vi "list energy peak.vi"() -> (1 "Energies Ordered":dbl[](array[numeric]), 2 "List Ordered":string[][](array[string]), 3 "List":string[][](array[string]))   [LabVIEW 2020]
uses:
  4b7d1e91-fce0-d643-892a-bcd5e833a70f.vi
  <vilib>/Utility/file.llb/Read Delimited Spreadsheet (string).vi
  <vilib>/Utility/Data Type/Get Array Information.vi
  <vilib>/Utility/Data Type/Get Type Information.vi
panel:
  out "appended array":string[][](array[string])
  out "list_peak_energies":string[][](array[string])
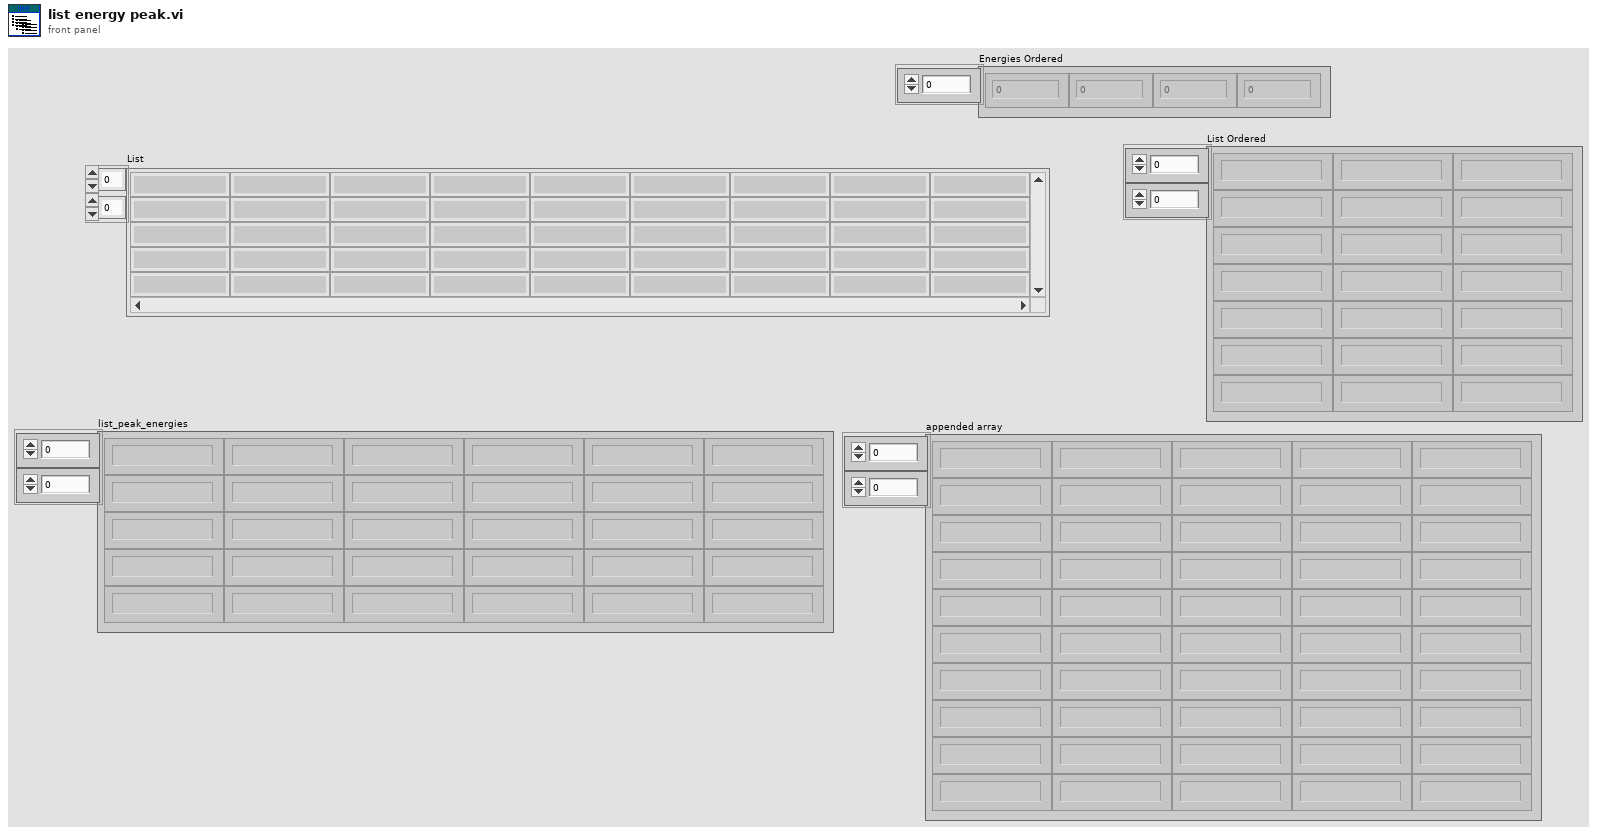
[diagram p1: front panel]
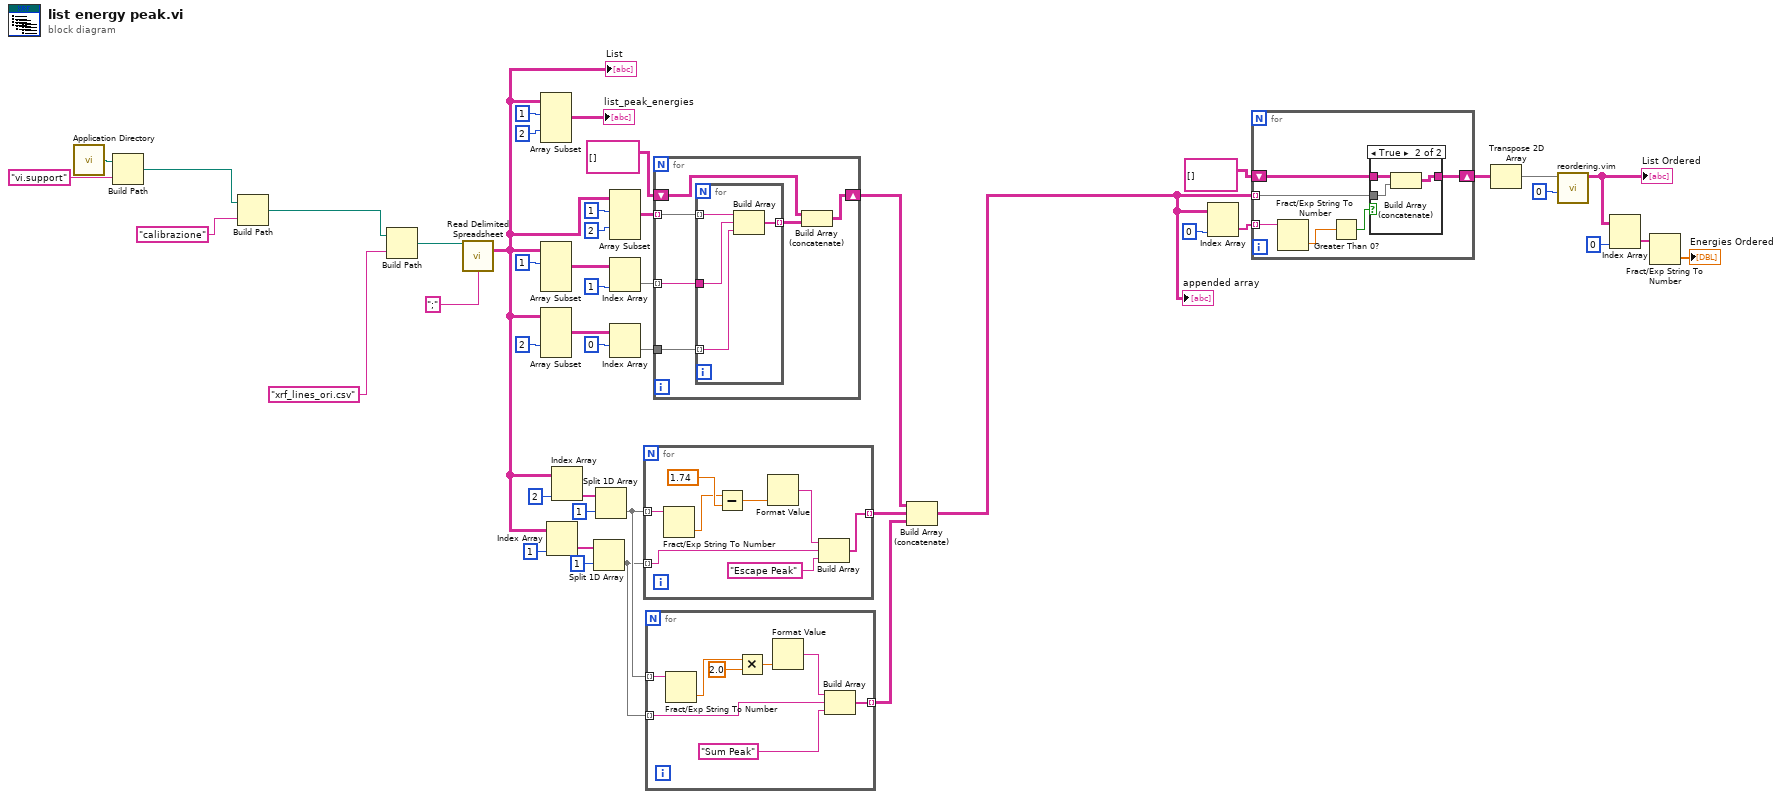
[diagram p0: block diagram]
diagram:
  n1 = call <vilib>:"Application Directory.vi"() -> ("Application Directory"=w40:path)
  n2 = Build Path(base path=w40, name or relative path="vi.support") -> (appended path=w3:path)
  n3 = Build Path(base path=w3, name or relative path="calibrazione") -> (appended path=w1:path)
  n4 = Build Path(base path=w1, name or relative path="xrf_lines_ori.csv") -> (appended path=w45:path)
  n5 = call-poly <vilib>:"Read Delimited Spreadsheet.vi"("file path (dialog if empty)"=w45, "delimiter (\\t)"=";" ("delimiter (\\t)")) -> ("all rows"=w12:string[][])  [unwired: 8 in, 5 out]
  "List" <- w12
  n6 = Array Subset(array=w12, index (row)=1 ("index"), index (col)=2 ("index")) -> (→"list_peak_energies":string[][])  [unwired: 2 in]
  n7 = Array Subset(array=w12, index (row)=1 ("index")) -> (w34:string[][])  [unwired: 3 in]
  n8 = Array Subset(array=w12, index (col)=2 ("index")) -> (w36:string[][])  [unwired: 3 in]
  n9 = Index Array(array=w12, index (col)=1 ("disabled index (col)")) -> (element=w14:string[])  [unwired: 1 in]
  n10 = Index Array(array=w12, index (col)=2 ("disabled index (col)")) -> (element=w10:string[])  [unwired: 1 in]
  n11 = Split 1D Array(array=w14, index=1) -> (second subarray=w8:string[])  [unwired: 1 out]
  n12 = Split 1D Array(array=w10, index=1) -> (second subarray=w9:string[])  [unwired: 1 out]
  n13 = Array Subset(array=w12, index (row)=1 ("index"), index (col)=2 ("index")) -> (w29:string[][])  [unwired: 2 in]
  n14 = Index Array(array=w34, index (col)=1 ("index (row)")) -> (element=w30:string[])  [unwired: 1 in]
  n15 = Index Array(array=w36, index (row)=0) -> (element=w31:string[])  [unwired: 1 in]
  n16 = for {
    tunnel: w9 -> [w54] mode=indexing
    tunnel: w8 -> [w47] mode=indexing
    tunnel: [w49] -> w7 mode=indexing
    n17 = Fract/Exp String To Number(string=w54) -> (number=w52:dbl)  [unwired: 3 in, 1 out]
    n18 = Subtract(x=w52, y=1.74) -> (x-y=w51:dbl)
    n19 = Format Value(value (0)=w51) -> (output string=w50:string)  [unwired: 2 in]
    n20 = Build Array(w50, w47, "Escape Peak") -> (w49:string[])
  }
  n21 = for {
    tunnel: w9 -> [w62] mode=indexing
    tunnel: w8 -> [w57] mode=indexing
    tunnel: [w55] -> w6 mode=indexing
    n22 = Fract/Exp String To Number(string=w62) -> (number=w60:dbl)  [unwired: 3 in, 1 out]
    n23 = Multiply(x=w60, y=2.0) -> (x*y=w59:dbl)
    n24 = Format Value(value (0)=w59) -> (output string=w58:string)  [unwired: 2 in]
    n25 = Build Array(w58, w57, "Sum Peak") -> (w55:string[])
  }
  n26 = for {
    tunnel: w29 -> [w66] mode=indexing
    tunnel: w31 -> [w68]
    tunnel: w30 -> [w67] mode=indexing
    shift-right: [w63] -> w5
    shift-left: string[][] [] -> [w64]
    n27 = for {
      tunnel: w68 -> [w71] mode=indexing
      tunnel: w67 -> [w72]
      tunnel: w66 -> [w69] mode=indexing
      tunnel: [w70] -> w65 mode=indexing
      n28 = Build Array(w69, w72, w71) -> (w70:string[])
    }
    n29 = Build Array (concatenate)(w64, w65) -> (w63:string[][])
  }
  n30 = Build Array (concatenate)(w5, w7, w6) -> (w4:string[][])
  "appended array" <- w4
  n31 = Index Array(array=w4, index (col)=0 ("disabled index (col)")) -> (element=w26:string[])  [unwired: 1 in]
  n32 = for {
    tunnel: w26 -> [w74] mode=indexing
    tunnel: w4 -> [w77] mode=indexing
    shift-right: [w75] -> w24
    shift-left: string[][] [] -> [w76]
    n33 = Fract/Exp String To Number(string=w74) -> (number=w73:dbl)  [unwired: 3 in, 1 out]
    n34 = Greater Than 0?(x=w73) -> (x > 0?=w78:bool)
    n35 = case shown="True" w78 {
      tunnel: w77 -> [_ w82]
      tunnel: w76 -> [w79 w81]
      tunnel: [w79 w80] -> w75
      frame False {
      }
      frame True {
        n36 = Build Array (concatenate)(w81, w82) -> (w80:string[][])
      }
    }
  }
  n37 = Transpose 2D Array(2D array=w24) -> (transposed array=w23:string[][])
  n38 = call "reordering.vim"("Row to Reorder"=0, "Data In"=w23) -> ("Data Out"=w20:string[][])  [unwired: 8 in, 1 out]
  "List Ordered" <- w20
  n39 = Index Array(array=w20, index (col)=0 ("disabled index (col)")) -> (element=w18:string[])  [unwired: 1 in]
  n40 = Fract/Exp String To Number(string=w18) -> (number=→"Energies Ordered":dbl[])  [unwired: 3 in, 1 out]
